vi "Example - Nested to Caller via interface.vi"   [LabVIEW 2023]
uses:
  Caller B/Caller B/Caller B.lvclass
  c:/dev/_r/4/eng/lv-core/lvpostprocessingd/lv_mc_x86_64/dist_i386/vi.lib/ActorFramework/Actor/Actor.lvclass
  Caller A/Caller A/Caller A.lvclass
  <vilib>/ActorFramework/Actor/Actor.lvclass
panel:
  # "Overview: This application demonstrates one of the uses of LabVIEW interfaces. It shows how an interface may be used to define an actor messaging interface. This allows a nested actor to talk to any caller actor that inherits from the interface. The nested actor avoids being tied to any single actor hierarchy.\n\nThis technique completely replaces the abstract message pattern used in LV 2019 and earlier.\n\nDetail: This VI launches two root actors, Caller A and Caller B. Each of those actors launches a nested actor. Those two nested actors are instances of the same class, Nested. Even though A and B have different parent classes, they both can receive messages from Nested. This same effect could be achieved without interfaces by putting methods on a common parent class, but a common parent class is not always an option. Also, each nested actor may have its own API requirements for its caller; using interfaces allows one caller to fulfill the requirements of multiple nested actors.\n\nNotice that the message class is not on Caller A or on Caller B but rather on Abstraction, the interface that both callers inherit. \n \nInstructions:\n1. Run this VI.\n2. Two windows will appear, one for Caller A and one for Caller B. Each button sends a message to that caller's Nested actor. Then Nested sends a response back, and the UI updates."
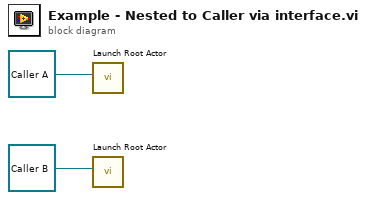
[diagram p0: block diagram]
diagram:
  n1 = call <vilib>:"Launch Root Actor.vi"("Actor"=refnum<class "Caller A.lvclass"> refnum ("Caller A.lvlib:Caller A.lvclass")) -> ()  [unwired: 9 in, 2 out]
  n2 = call <vilib>:"Launch Root Actor.vi"("Actor"=refnum<class "Caller B.lvclass"> refnum ("Caller B.lvlib:Caller B.lvclass")) -> ()  [unwired: 9 in, 2 out]
